vi "Framework.Offset Inline Buffers.vi"(8 "error in (no error)":errorcluster, 11 "Framework in":refnum<class "Framework.lvclass">) -> (0 "error out":errorcluster, 3 "Framework out":refnum<class "Framework.lvclass">)   [LabVIEW 2017, in "DSF Core.lvlib" / "Framework.lvclass"]
uses:
  Framework.lvclass
  Framework.lvclass/Framework.ctl
  Plugin/Plugin.lvclass
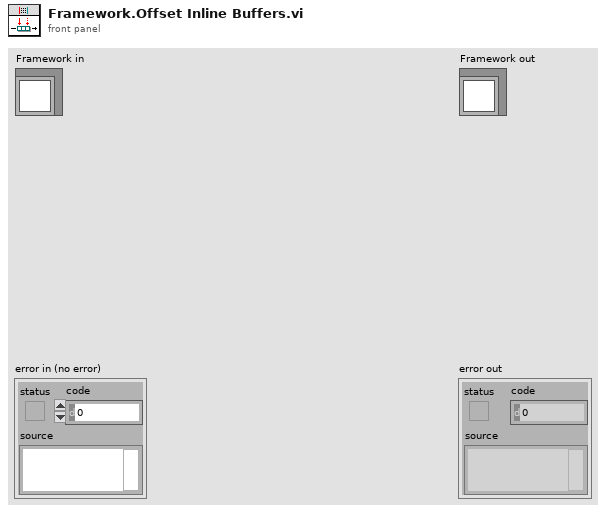
[diagram p1: front panel]
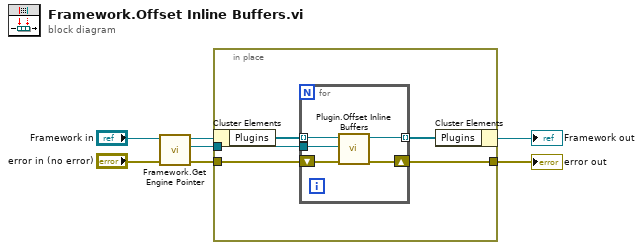
[diagram p0: block diagram]
diagram:
  n1 = call "Framework.Get Engine Pointer.vi"("Framework in"="Framework in") -> ("Engine Pointer"=w1:refnum<class "Memory.Pointer.lvclass">, "Framework out"=w2:refnum<class "Framework.lvclass">)  [unwired: 9 in]
  n2 = in-place {
    in-place-border: "error in (no error)" -> [w8]
    in-place-border: [w9] -> w5
    in-place-border: w1 -> [w7]
    n3 = in-place-cluster #1(w2) -> ("Plugins"=w11:refnum<class "Plugin.lvclass">[])
    n4 = for {
      tunnel: w11 -> [w16] mode=indexing
      tunnel: [w15] -> w10 mode=indexing
      shift-right: [w14] -> w9
      shift-left: w8 -> [w13]
      tunnel: w7 -> [w12]
      n5 = call "Plugin.Offset Inline Buffers.vi"("error in (no error)"=w13, "Engine Pointer"=w12, "Plugin in"=w16) -> ("error out"=w14:errorcluster, "Plugin out"=w15:refnum<class "Plugin.lvclass">)  [unwired: 7 in]
    }
    n6 = in-place-cluster #1("Plugins"=w10) -> (→"Framework out":refnum<class "Framework.lvclass">)
  }
  "error out" <- w5
